vi "Edit_BSA_setup.vi"(1 "BSA info":T1={"GPIB Address"="13", "No of Check Bytes"=4, "Extra Info"="57N11", "COLOUR"=52224, "Wavelength (nm)"=52224.0} {"Wavelength (nm)" format="%.1f"}, 3 "BSA 1?":bool, 7 "Multiply Velocity by -1":bool) -> (4 "Centre frequency":dbl format="%.2f", 5 "Bandwidth":dbl format="%.2f", 6 "Output":T5={"Output data format"=enum."Velocity", "Non-validated signals"=enum."Reject"}, 9 "Calibration factor":dbl=3.97 format="%.4f", 10 "Signal conditioning (out)":T6={"High voltage"=2000, "Signal gain (dB)"=45} {"Signal gain (dB)" min=0 max=57 step=1; "High voltage" min=0 max=2040 step=8}, 11 "Buffer mode out":enum16{"One shot", "Ring", "FIFO"}(ring), 12 "Anode current limit (mA)":T8(ring), 14 "Range (out)":T7={"Centre frequency"=16, "Bandwidth"=10, "Units"=enum."m/s", "Frequency shift"=enum."Enabled"} {"Bandwidth" items=["3.776E-3", "7.553E-3", "15.105E-3", "30.211E-3", "60.422E-3", "120.844E-3", "241.687E-3", "483.375E-3", "966.750E-3", "1.933E+0", "3.867E+0", "7.734E+0", "15.468E+0", "30.936E+0"]; "Centre frequency" items=["-15.468E+0", "-14.501E+0", "-13.534E+0", "-12.568E+0", "-11.601E+0", "-10.634E+0", "-9.667E+0", "-8.701E+0", "-7.734E+0", "-6.767E+0", "-5.800E+0", "-4.834E+0", "-3.867E+0", "-2.900E+0", "-1.933E+0", "-966.750E-3", "0.000E+0", "966.750E-3", "1.933E+0", "2.900E+0", "3.867E+0", "4.834E+0", "5.800E+0", "6.767E+0", "7.734E+0", "8.701E+0", "9.667E+0", "10.634E+0", "11.601E+0", "12.568E+0", "13.534E+0", "14.501E+0", "15.468E+0"]}, 15 "Selected range":cluster{"Minimum":dbl, "Maximum":dbl}={"Minimum"=-1.9850000000000005, "Maximum"=1.9850000000000005} {"Maximum" format="%.2f"; "Minimum" format="%.2f"}, 17 "Clock parameters (out)":T2={"Arrival time clock"=enum."Internal", "Clock source"=enum."Private", "Coincidence"=enum."Master"}, 18 "Data collection mode (out)":T4 {"Duty cycle (%)" format="%.2f"; "Dead time (s)" format="%.2f"}, 19 "Analysis parameters (out)":T3={"Burst criterion"=enum."Envelope", "Oversize reject level"=enum."1 (disabled)", "Pedestal attenuation"=enum."0", "Record length"=enum."16", "Quality factor"=0} {"Quality factor" min=0 max=80 step=10})   [LabVIEW 2011]
uses:
  Controls/ok_button.ctl
  Controls/BSA_info_Cluster.ctl
  Globals/LDA_meas_global_1.vi
  Globals/LDA_meas_global_2.vi
panel:
  out "45 Degree Mirror":bool
  in  "Component":string="W"
  out "error out":errorcluster
  in  "Clock parameters":T2={"Arrival time clock"=enum."Internal", "Clock source"=enum."Private", "Coincidence"=enum."Master"}
  in  "Analysis parameters":T3={"Burst criterion"=enum."Envelope", "Oversize reject level"=enum."1 (disabled)", "Pedestal attenuation"=enum."0", "Record length"=enum."16", "Quality factor"=0} {"Quality factor" min=0 max=80 step=10}
  in  "Data collection mode":T4 {"Duty cycle (%)" format="%.2f"; "Dead time (s)" format="%.2f"}
  in  "Buffer mode":enum16{"One shot", "Ring", "FIFO"}(ring)
  in  "OK":T9
  in  "Signal conditioning":T6={"High voltage"=1600, "Signal gain (dB)"=35} {"Signal gain (dB)" min=0 max=57 step=1; "High voltage" min=0 max=1600 step=8}
  in  "Range":T10={"Centre Velocity"=16, "Velocity span"=10, "Units"=enum."m/s", "Frequency shift"=enum."Enabled"} {"Velocity span" items=["3.582E-3", "7.164E-3", "14.328E-3", "28.656E-3", "57.312E-3", "114.625E-3", "229.250E-3", "458.500E-3", "917.000E-3", "1.834E+0", "3.668E+0", "7.336E+0", "14.672E+0", "29.344E+0"]; "Centre Velocity" items=["-7.336E+0", "-6.877E+0", "-6.419E+0", "-5.960E+0", "-5.502E+0", "-5.043E+0", "-4.585E+0", "-4.127E+0", "-3.668E+0", "-3.209E+0", "-2.751E+0", "-2.292E+0", "-1.834E+0", "-1.375E+0", "-917.000E-3", "-458.500E-3", "0.000E+0", "458.500E-3", "917.000E-3", "1.375E+0", "1.834E+0", "2.292E+0", "2.751E+0", "3.209E+0", "3.668E+0", "4.127E+0", "4.585E+0", "5.043E+0", "5.502E+0", "5.960E+0", "6.419E+0", "6.877E+0", "7.336E+0"]}
  # "These values can be\nchanged in LDA Setup\nrun from the EnFlo Hub"
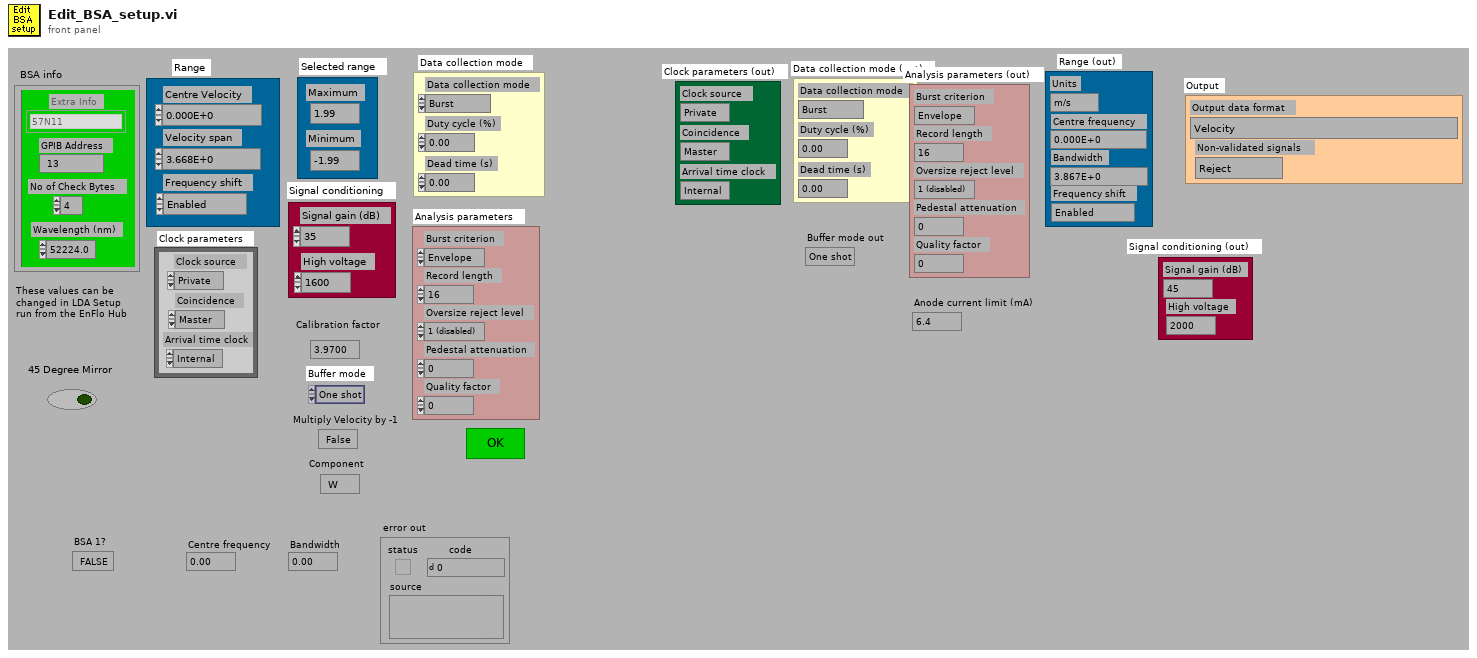
[diagram p1: front panel]
types:
  T1 = typedef "BSA_info_Cluster.ctl" = cluster{"GPIB Address":string, "No of Check Bytes":i32, "Extra Info":string, "COLOUR":u32, "Wavelength (nm)":dbl}
  T2 = cluster{"Arrival time clock":enum16{"External", "Internal"}, "Clock source":enum16{"Slave", "Master", "Private"}, "Coincidence":enum16{"Slave", "Master", "Private"}}
  T3 = cluster{"Burst criterion":enum16{"Envelope", "Pedestal", "Env and ped"}, "Oversize reject level":enum16{"1 (disabled)", "2", "3", "4", "5", "6", "7", "8", "9"}, "Pedestal attenuation":enum16{"0", "6", "12", "18"}, "Record length":enum16{"8", "16", "32", "64"}, "Quality factor":i16}
  T4 = cluster{"Dead time (s)":dbl, "Duty cycle (%)":dbl, "Data collection mode":enum16{"Burst", "Contiuous", "Dead time", "External"}}
  T5 = cluster{"Output data format":enum16{"Velocity, transit time, arrival time", "Velocity, arrival time", "Velocity, transit time", "Velocity"}, "Non-validated signals":enum16{"Accept", "Reject"}}
  T6 = cluster{"High voltage":i16, "Signal gain (dB)":i16}
  T7 = cluster{"Centre frequency":u16, "Bandwidth":u16, "Units":enum16{"Hz", "m/s"}, "Frequency shift":enum16{"Disabled", "Enabled"}}
  T8 = enum16{"6.4", "3.2", "1.6", "0.8", "0.4", "0.2", "0.1", "0.05"}
  T9 = typedef "ok_button.ctl" = bool
  T10 = cluster{"Centre Velocity":u16, "Velocity span":u16, "Units":enum16{"Hz", "m/s"}, "Frequency shift":enum16{"Disabled", "Enabled"}}
  T11 = enum16{"Burst", "Contiuous", "Dead time", "External"}
  T12 = enum16{"1 (disabled)", "2", "3", "4", "5", "6", "7", "8", "9"}
  T13 = enum16{"Velocity, transit time, arrival time", "Velocity, arrival time", "Velocity, transit time", "Velocity"}
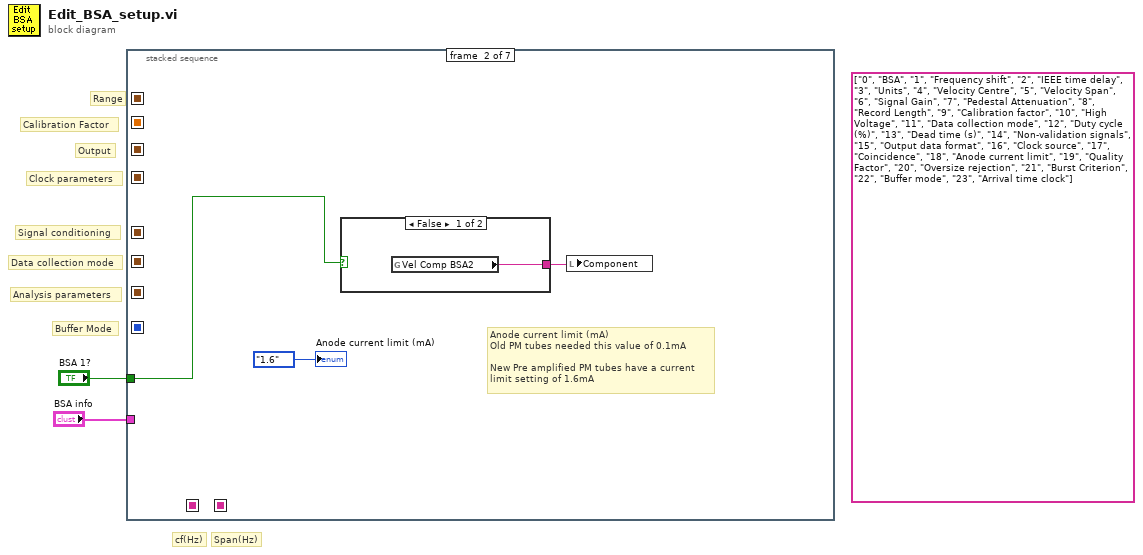
[diagram p0: block diagram]
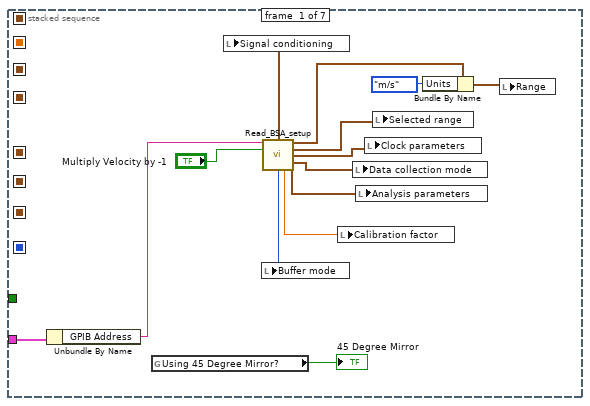
[diagram p2: hidden frame]
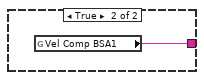
[diagram p3: hidden frame]
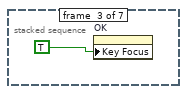
[diagram p4: hidden frame]
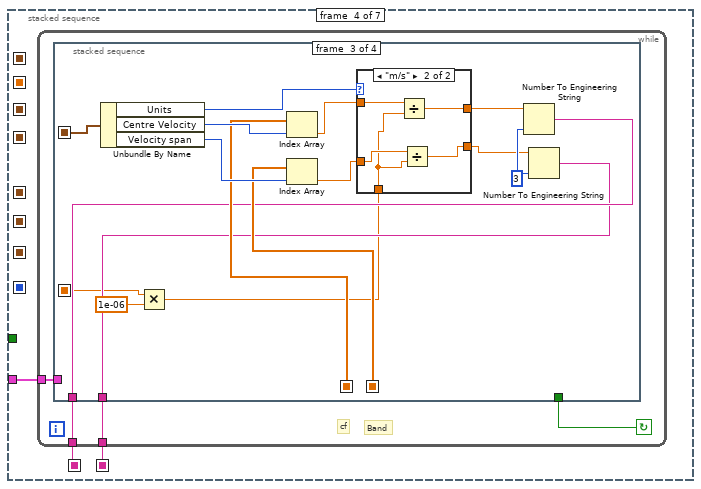
[diagram p5: hidden frame]
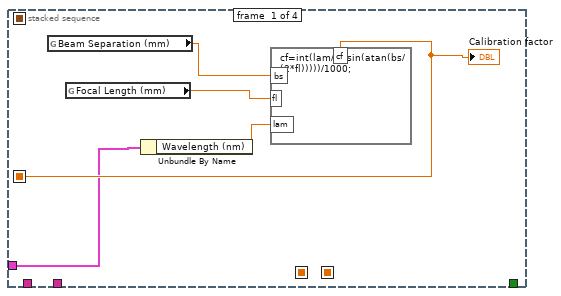
[diagram p6: hidden frame]
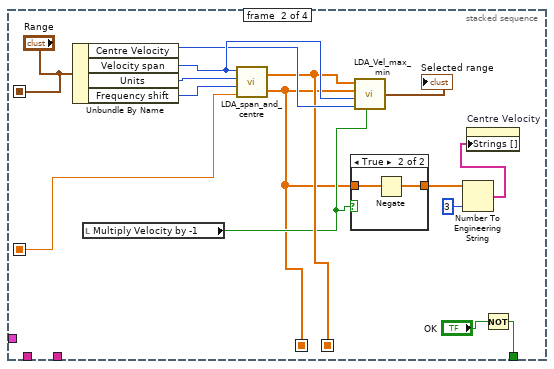
[diagram p7: hidden frame]
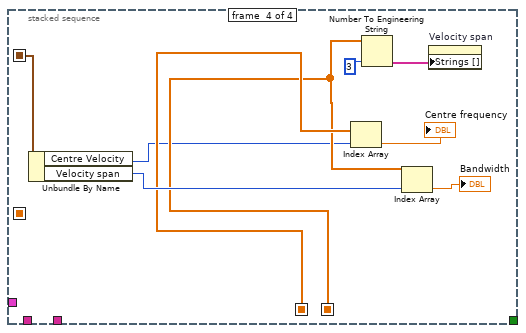
[diagram p10: hidden frame]
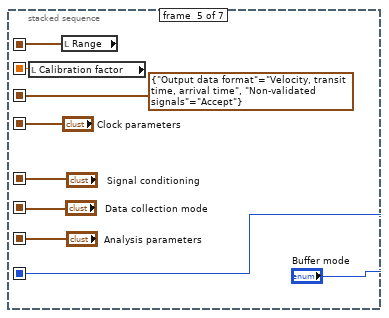
[diagram p11: hidden frame]
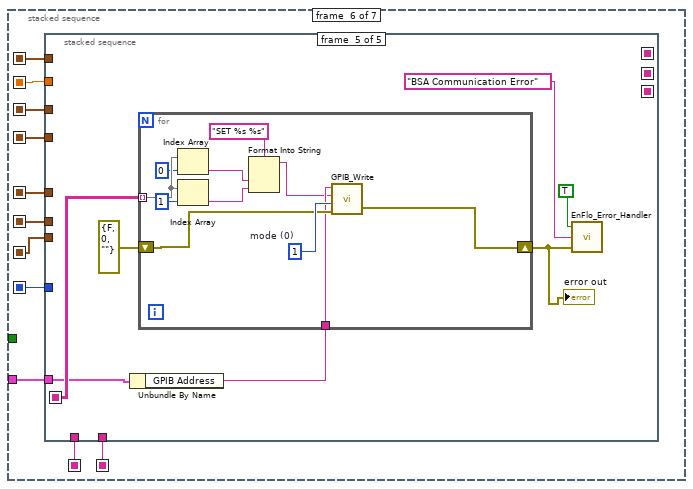
[diagram p12: hidden frame]
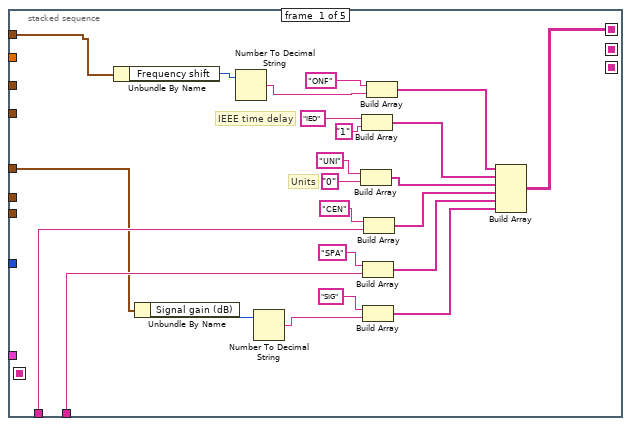
[diagram p13: hidden frame]
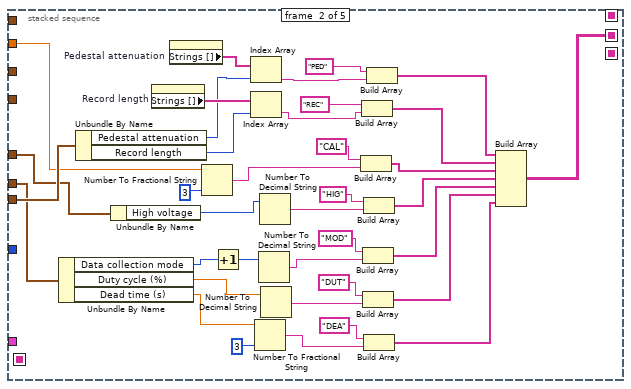
[diagram p14: hidden frame]
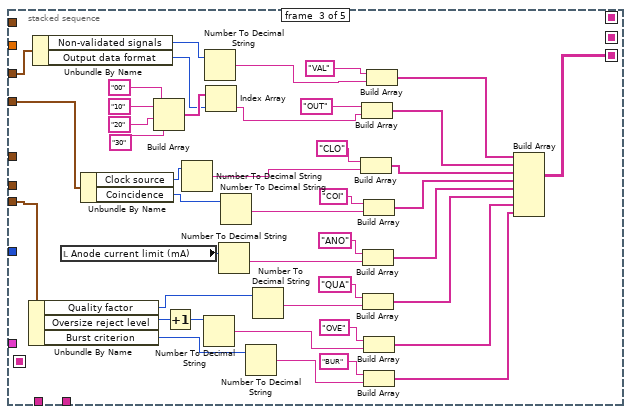
[diagram p15: hidden frame]
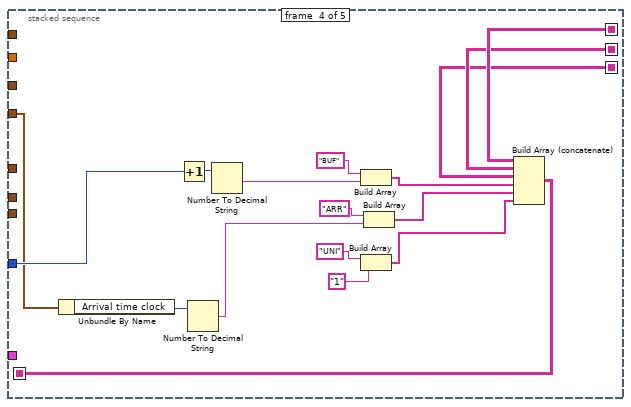
[diagram p16: hidden frame]
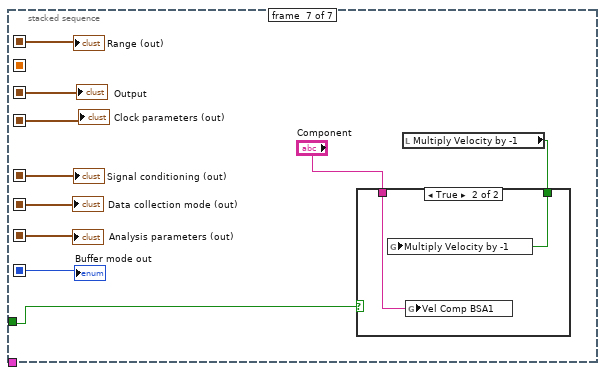
[diagram p17: hidden frame]
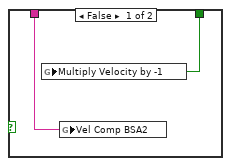
[diagram p18: hidden frame]
diagram:
  (unwired) string[][] [["0", "BSA"], ["1", "Frequency shift"], ["2", "IEEE time delay"], ["3", "Units"], ["4", "Velocity Centre"], ["5", "Velocity Span"], ["6", "Signal Gain"], ["7", "Pedestal Attenuation"], ["8", "Record Length"], ["9", "Calibration factor"], ["10", "High Voltage"], ["11", "Data collection mode"], ["12", "Duty cycle (%)"], ["13", "Dead time (s)"], ["14", "Non-validation signals"], ["15", "Output data format"], ["16", "Clock source"], ["17", "Coincidence"], ["18", "Anode current limit"], ["19", "Quality Factor"], ["20", "Oversize rejection"], ["21", "Burst Criterion"], ["22", "Buffer mode"], ["23", "Arrival time clock"]]
  # "Span(Hz)"
  # "cf(Hz)"
  # "Buffer Mode"
  # "Clock parameters"
  # "Output"
  # "Calibration Factor"
  # "Data collection mode"
  # "Analysis parameters"
  # "Signal conditioning"
  # "Range"
  n1 = stacked-sequence {
    seq-local: [_ _ _ _ w89 _ _] -> [_ _ _ _ _ w103 w250]
    seq-local: [_ _ _ _ w90 _ _] -> [_ _ _ _ _ w98 _]
    seq-local: [_ _ _ _ T5 {"Output data format"=enum."Velocity, transit time, arrival time", "Non-validated signals"=enum."Accept"} ("Output") _ _] -> [_ _ _ _ _ w96 w245]
    seq-local: [_ _ _ _ "Clock parameters" _ _] -> [_ _ _ _ _ w95 w246]
    seq-local: [_ _ _ _ "Signal conditioning" _ _] -> [_ _ _ _ _ w100 w247]
    seq-local: [_ _ _ _ "Data collection mode" _ _] -> [_ _ _ _ _ w97 w249]
    seq-local: [_ _ _ _ "Analysis parameters" _ _] -> [_ _ _ _ _ w99 w248]
    seq-local: [_ _ _ _ "Buffer mode" _ _] -> [_ _ _ _ _ w94 w241]
    seq-local: [_ _ _ w25 _ _ _] -> [_ _ _ _ _ w102 _]
    seq-local: [_ _ _ w24 _ _ _] -> [_ _ _ _ _ w101 _]
    tunnel: "BSA 1?" -> [_ w17 _ _ _ _ w244]
    tunnel: "BSA info" -> [w5 _ _ w23 _ w93 _]
    frame #0 {
      n2 = Unbundle By Name(w5) -> ("GPIB Address"=w4:string)
      n3 = global read "LDA_meas_global_1.vi" "Using 45 Degree Mirror?"() -> (→"45 Degree Mirror":bool)
      n4 = call "Read_BSA_setup.vi"("GPIB Address"=w4, "Multiply Velocity by -1"="Multiply Velocity by -1") -> ("Signal conditioning"=w16:T6, "Range"=w9:T10, "Selected range"=w10:cluster{"Minimum":dbl, "Maximum":dbl}, "Clock parameters"=w11:T2, "Data collection mode"=w12:T4, "Buffer mode"=w15:enum16{"One shot", "Ring", "FIFO"}, "Calibration factor"=w14:dbl, "Analysis parameters"=w13:T3)  [unwired: 1 in, 5 out]
      n5 = local write "Signal conditioning"(w16) -> ()
      n6 = local write "Buffer mode"(w15) -> ()
      n7 = local write "Calibration factor"(w14) -> ()
      n8 = local write "Data collection mode"(w12) -> ()
      n9 = local write "Analysis parameters"(w13) -> ()
      n10 = local write "Clock parameters"(w11) -> ()
      n11 = local write "Selected range"(w10) -> ()
      n12 = Bundle By Name(cluster=w9, "Units"=enum16{"Hz", "m/s"}."m/s") -> (w8:T10)
      n13 = local write "Range"(w8) -> ()
    }
    frame #1 {
      # "Anode current limit (mA)\nOld PM tubes needed this value of 0.1mA\n\nNew Pre amplified PM tubes have a current\nlimit setting of 1.6mA"
      n14 = case shown="False" w17 {
        tunnel: [w20 w21] -> w18
        frame False {
          n15 = global read "LDA_meas_global_2.vi" "Vel Comp BSA2"() -> (w20:string)
        }
        frame True {
          n16 = global read "LDA_meas_global_1.vi" "Vel Comp BSA1"() -> (w21:string)
        }
      }
      n17 = local write "Component"(w18) -> ()
      "Anode current limit (mA)" <- T8."1.6" ("Anode current limit (mA)")
    }
    frame #2 {
      n18 = property on="OK" class="Bool"("Key Focus"=TRUE ("Visible")) -> ()  [unwired: 2 in, 2 out]
    }
    frame #3 {
      n19 = while {
        tunnel: [w27] -> w24
        tunnel: [w28] -> w25
        tunnel: w23 -> [w26]
        stop <- w29 continue-if-true
        # "Band"
        # "cf"
        n20 = stacked-sequence {
          seq-local: [w31 _ _ _] -> [_ w35 w60 _]
          seq-local: [_ w36 _ _] -> [_ _ w64 w80]
          seq-local: [_ w41 _ _] -> [_ _ w63 w79]
          seq-local: [_ "Range" _ _] -> [_ _ w68 w84]
          tunnel: [_ w48 _ _] -> w29
          tunnel: [_ _ w62 _] -> w28
          tunnel: [_ _ w61 _] -> w27
          tunnel: w26 -> [w30 _ _ _]
          frame #0 {
            n21 = global read "LDA_meas_global_1.vi" "Beam Separation (mm)"() -> (w33:dbl)
            n22 = global read "LDA_meas_global_1.vi" "Focal Length (mm)"() -> (w32:dbl)
            n23 = Unbundle By Name(w30) -> ("Wavelength (nm)"=w34:dbl)
            n24 = formula code="cf=int(lam/2/(sin(atan(bs/(2*fl)))))/1000;"("bs"=w33, "fl"=w32, "lam"=w34) -> ("cf"=w31:dbl)
            "Calibration factor" <- w31
          }
          frame #1 {
            n25 = Unbundle By Name("Range") -> ("Centre Velocity"=w43:u16, "Velocity span"=w44:u16, "Units"=w46:enum16{"Hz", "m/s"}, "Frequency shift"=w45:enum16{"Disabled", "Enabled"})
            n26 = local read "Multiply Velocity by -1"() -> (w40:bool)
            n27 = call "LDA_span_and_centre.vi"("Calibration factor"=w35, "Frequency shift"=w45, "Units"=w46, "Velocity span"=w44) -> ("Centres"=w36:dbl[], "Spans"=w41:dbl[])
            n28 = case shown="True" w40 {
              tunnel: [w50 w51] -> w37
              tunnel: w36 -> [w50 w52]
              frame False {
              }
              frame True {
                n29 = Negate(x=w52) -> (-x=w51:dbl[])
              }
            }
            n30 = call "LDA_Vel_max_min.vi"("Multiply Velocity by -1"=w40, "Centre Velocity"=w43, "Velocity span"=w44, "Centres"=w36, "Spans"=w41) -> ("Selected range"=→"Selected range":cluster{"Minimum":dbl, "Maximum":dbl})  [unwired: 1 out]
            n31 = Number To Engineering String(2:i16 3 ("precision (6)"), 4:w37) -> (0:w38:string[])  [unwired: 2 out]
            n32 = property on="Centre Velocity" class="Ring (strict)"("Strings []"=w38) -> ()  [unwired: 2 in, 2 out]
            n33 = Not(x="OK") -> (.not. x?=w48:T9)
          }
          frame #2 {
            w65 = 3
            n34 = Unbundle By Name(w68) -> ("Units"=w55:enum16{"Hz", "m/s"}, "Centre Velocity"=w66:u16, "Velocity span"=w67:u16)
            n35 = Multiply(x=w60, y=1e-06) -> (x*y=w58:dbl)
            n36 = Index Array(array=w64, index=w66) -> (element=w56:dbl)
            n37 = Index Array(array=w63, index=w67) -> (element=w57:dbl)
            n38 = case shown="\"m/s\"" w55 {
              tunnel: w56 -> [w70 w75]
              tunnel: [w70 w71] -> w54
              tunnel: w57 -> [w69 w74]
              tunnel: [w69 w72] -> w53
              tunnel: w58 -> [_ w73]
              frame "Hz" {
              }
              frame "m/s" {
                n39 = Divide(x=w75, y=w73) -> (x/y=w71:dbl)
                n40 = Divide(x=w74, y=w73) -> (x/y=w72:dbl)
              }
            }
            n41 = Number To Engineering String(2:w65, 4:w54) -> (0:w62:string)  [unwired: 2 out]
            n42 = Number To Engineering String(2:w65, 4:w53) -> (0:w61:string)  [unwired: 2 out]
          }
          frame #3 {
            n43 = Unbundle By Name(w84) -> ("Centre Velocity"=w77:u16, "Velocity span"=w81:u16)
            n44 = Index Array(array=w80, index=w77) -> (element=→"Centre frequency":dbl)
            n45 = Number To Engineering String(2:3, 4:w79) -> (0:w78:string[])  [unwired: 2 out]
            n46 = Index Array(array=w79, index=w81) -> (element=→"Bandwidth":dbl)
            n47 = property on="Velocity span" class="Ring (strict)"("Strings []"=w78) -> ()  [unwired: 2 in, 2 out]
          }
        }
      }
    }
    frame #4 {
      n48 = local read "Calibration factor"() -> (w90:dbl)
      n49 = local read "Range"() -> (w89:T10)
    }
    frame #5 {
      n50 = stacked-sequence {
        seq-local: [w104 _ _ _ _] -> [_ _ _ w212 _]
        seq-local: [_ w127 _ _ _] -> [_ _ _ w211 _]
        seq-local: [_ _ w164 _ _] -> [_ _ _ w210 _]
        seq-local: [_ _ _ w209 _] -> [_ _ _ _ w229]
        tunnel: w103 -> [w126 _ _ _ _]
        tunnel: w102 -> [w117 _ _ _ _]
        tunnel: w101 -> [w115 _ _ _ _]
        tunnel: w100 -> [w112 w141 _ _ _]
        tunnel: w99 -> [_ w149 w173 _ _]
        tunnel: w98 -> [_ w143 _ _ _]
        tunnel: w97 -> [_ w138 _ _ _]
        tunnel: w96 -> [_ _ w191 _ _]
        tunnel: w95 -> [_ _ w181 w215 _]
        tunnel: w94 -> [_ _ _ w217 _]
        tunnel: w93 -> [_ _ _ _ w225]
        frame #0 {
          # "Units"
          # "IEEE time delay"
          n51 = Unbundle By Name(w126) -> ("Frequency shift"=w125:enum16{"Disabled", "Enabled"})
          n52 = Unbundle By Name(w112) -> ("Signal gain (dB)"=w113:i16)
          n53 = Number To Decimal String(number=w125) -> (decimal integer string=w123:string)  [unwired: 1 out]
          n54 = Number To Decimal String(number=w113) -> (decimal integer string=w111:string)  [unwired: 1 out]
          n55 = Build Array("UNI", "0") -> (w108:string[])
          n56 = Build Array("IED", "1" ("element")) -> (w109:string[])
          n57 = Build Array("SPA", w115) -> (w106:string[])
          n58 = Build Array("SIG", w111) -> (w105:string[])
          n59 = Build Array("CEN", w117) -> (w107:string[])
          n60 = Build Array("ONF", w123) -> (w110:string[])
          n61 = Build Array(w110, w109, w108, w107, w106, w105) -> (w104:string[][])
        }
        frame #1 {
          n62 = Unbundle By Name(w138) -> ("Data collection mode"=w133:T11, "Duty cycle (%)"=w132:dbl, "Dead time (s)"=w131:dbl)
          n63 = Unbundle By Name(w149) -> ("Pedestal attenuation"=w148:enum16{"0", "6", "12", "18"}, "Record length"=w147:enum16{"8", "16", "32", "64"})
          n64 = Unbundle By Name(w141) -> ("High voltage"=w140:i16)
          n65 = property on="Record length" class="Enum (strict)"() -> ("Strings []"=w150:string[])  [unwired: 2 in, 2 out]
          n66 = property on="Pedestal attenuation" class="Enum (strict)"() -> ("Strings []"=w151:string[])  [unwired: 2 in, 2 out]
          n67 = Number To Fractional String(number=w143, precision (6)=3) -> (F-format string=w142:string)  [unwired: 2 out]
          n68 = Increment(x=w133) -> (x+1=w136:T11)
          n69 = Index Array(array=w151, index=w148) -> (element=w145:string)
          n70 = Index Array(array=w150, index=w147) -> (element=w146:string)
          n71 = Number To Fractional String(number=w131, precision (6)=3) -> (F-format string=w130:string)  [unwired: 2 out]
          n72 = Number To Decimal String(number=w136) -> (decimal integer string=w128:string)  [unwired: 1 out]
          n73 = Number To Decimal String(number=w140) -> (decimal integer string=w139:string)  [unwired: 1 out]
          n74 = Number To Decimal String(number=w132) -> (decimal integer string=w129:string)  [unwired: 1 out]
          n75 = Build Array("CAL", w142) -> (w155:string[])
          n76 = Build Array("REC", w146) -> (w156:string[])
          n77 = Build Array("MOD", w128) -> (w153:string[])
          n78 = Build Array("DUT", w129) -> (w152:string[])
          n79 = Build Array("HIG", w139) -> (w154:string[])
          n80 = Build Array("DEA", w130) -> (w134:string[])
          n81 = Build Array("PED", w145) -> (w157:string[])
          n82 = Build Array(w157, w156, w155, w154, w153, w152, w134) -> (w127:string[][])
        }
        frame #2 {
          n83 = Unbundle By Name(w173) -> ("Quality factor"=w171:i16, "Oversize reject level"=w170:T12, "Burst criterion"=w169:enum16{"Envelope", "Pedestal", "Env and ped"})
          n84 = Unbundle By Name(w191) -> ("Non-validated signals"=w185:enum16{"Accept", "Reject"}, "Output data format"=w184:T13)
          n85 = local read "Anode current limit (mA)"() -> (w176:T8)
          n86 = Unbundle By Name(w181) -> ("Clock source"=w180:enum16{"Slave", "Master", "Private"}, "Coincidence"=w179:enum16{"Slave", "Master", "Private"})
          n87 = Build Array("00", "10", "20", "30") -> (w186:string[])
          n88 = Increment(x=w170) -> (x+1=w172:T12)
          n89 = Number To Decimal String(number=w180) -> (decimal integer string=w178:string)  [unwired: 1 out]
          n90 = Number To Decimal String(number=w172) -> (decimal integer string=w167:string)  [unwired: 1 out]
          n91 = Number To Decimal String(number=w185) -> (decimal integer string=w183:string)  [unwired: 1 out]
          n92 = Index Array(array=w186, index=w184) -> (element=w182:string)
          n93 = Number To Decimal String(number=w176) -> (decimal integer string=w175:string)  [unwired: 1 out]
          n94 = Number To Decimal String(number=w179) -> (decimal integer string=w177:string)  [unwired: 1 out]
          n95 = Number To Decimal String(number=w169) -> (decimal integer string=w168:string)  [unwired: 1 out]
          n96 = Number To Decimal String(number=w171) -> (decimal integer string=w166:string)  [unwired: 1 out]
          n97 = Build Array("CLO", w178) -> (w197:string[])
          n98 = Build Array("OUT", w182) -> (w198:string[])
          n99 = Build Array("ANO", w175) -> (w195:string[])
          n100 = Build Array("QUA", w166) -> (w194:string[])
          n101 = Build Array("COI", w177) -> (w196:string[])
          n102 = Build Array("OVE", w167) -> (w192:string[])
          n103 = Build Array("BUR", w168) -> (w165:string[])
          n104 = Build Array("VAL", w183) -> (w199:string[])
          n105 = Build Array(w199, w198, w197, w196, w195, w194, w192, w165) -> (w164:string[][])
        }
        frame #3 {
          n106 = Unbundle By Name(w215) -> ("Arrival time clock"=w214:enum16{"External", "Internal"})
          n107 = Increment(x=w217) -> (x+1=w218:enum16{"One shot", "Ring", "FIFO"})
          n108 = Number To Decimal String(number=w214) -> (decimal integer string=w213:string)  [unwired: 1 out]
          n109 = Number To Decimal String(number=w218) -> (decimal integer string=w216:string)  [unwired: 1 out]
          n110 = Build Array("BUF", w216) -> (w220:string[])
          n111 = Build Array("UNI", "1" ("element")) -> (w206:string[])
          n112 = Build Array("ARR", w213) -> (w219:string[])
          n113 = Build Array (concatenate)(w212, w211, w210, w220, w219, w206) -> (w209:string[][])
        }
        frame #4 {
          n114 = Unbundle By Name(w225) -> ("GPIB Address"=w224:string)
          n115 = for {
            tunnel: w229 -> [w236] mode=indexing
            shift-right: [w239] -> w223
            shift-left: errorcluster {"status"=FALSE, "code"=0, "source"=""} ("error out") -> [w238]
            tunnel: w224 -> [w237]
            w240 = i16 1  # mode (0)
            n116 = Index Array(array=w236, index=0) -> (element=w233:string)
            n117 = Index Array(array=w236, index=1) -> (element=w232:string)
            n118 = Format Into String(format string="SET %s %s", w233, w232) -> (resulting string=w230:string)  [unwired: 2 in, 1 out]
            n119 = call "GPIB_Write.vi"("address string"=w237, "data In"=w230, "mode (0)"=w240, "error in"=w238) -> ("error out"=w239:errorcluster)  [unwired: 1 in, 1 out]
          }
          "error out" <- w223
          n120 = call "EnFlo_Error_Handler.vi"("error in (no error)"=w223, "Error Type"="BSA Communication Error", "Dialog Box (T)"=TRUE) -> ()  [unwired: 3 out]
        }
      }
    }
    frame #6 {
      n121 = local read "Multiply Velocity by -1"() -> (w242:bool)
      n122 = case shown="True" w244 {
        tunnel: "Component" -> [w252 w254]
        tunnel: w242 -> [w251 w253]
        frame False {
          n123 = global write "LDA_meas_global_2.vi" "Multiply Velocity by -1"(w251) -> ()
          n124 = global write "LDA_meas_global_2.vi" "Vel Comp BSA2"(w252) -> ()
        }
        frame True {
          n125 = global write "LDA_meas_global_1.vi" "Multiply Velocity by -1"(w253) -> ()
          n126 = global write "LDA_meas_global_1.vi" "Vel Comp BSA1"(w254) -> ()
        }
      }
      "Range (out)" <- w250
      "Signal conditioning (out)" <- w247
      "Analysis parameters (out)" <- w248
      "Output" <- w245
      "Clock parameters (out)" <- w246
      "Data collection mode (out)" <- w249
      "Buffer mode out" <- w241
    }
  }
